vi "Py - Cs Total loop.vi"(6 "rho":dbl, 7 "python in":refnum<k35>, 8 "error in":errorcluster, 9 "Int_array":dbl[](array[numeric]), 10 "En_array":dbl[](array[numeric]), 11 "Z":i32) -> (0 "error out":errorcluster, 3 "Cs Total":dbl, 5 "python out":refnum<k35>)   [LabVIEW 2023]
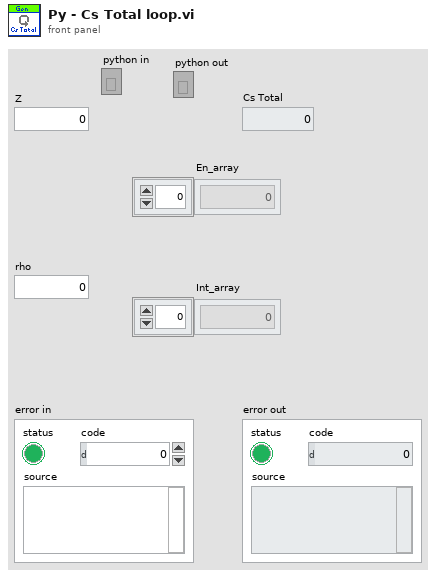
[diagram p1: front panel]
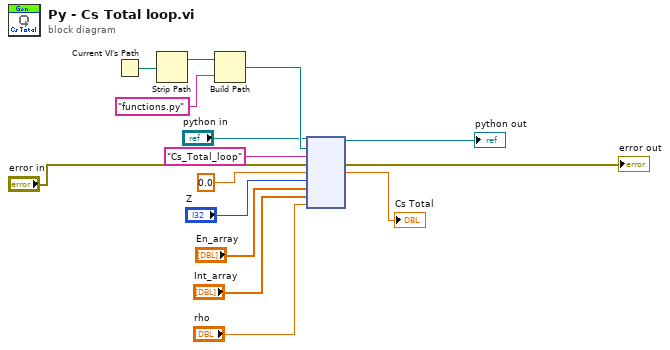
[diagram p0: block diagram]
diagram:
  n1 = Current VI's Path() -> (path=w14:path)
  n2 = Strip Path(path=w14) -> (stripped path=w13:path)  [unwired: 1 out]
  n3 = Build Path(base path=w13, name or relative path="functions.py") -> (appended path=w9:path)
  n4 = node("python in", w9, "Cs_Total_loop", "error in", 0.0, "Z", "En_array", "Int_array", "rho") -> (→"python out":refnum<k35>, →"error out":errorcluster, →"Cs Total":dbl)  [unwired: 4 in, 2 out]
